vi "User Event LV2 Stop.vi"(0 "Stop":bool=TRUE, 11 "Error In":errorcluster, 13 "Operation":T1) -> (4 "User Event Ref":refnum<user-event>, 15 "Error Out":errorcluster)   [LabVIEW 2023]
doc: "The file is the Functional global to store the user event reference to stop when user clicks panel close."
uses:
  Typedef/User Event Operations.ctl
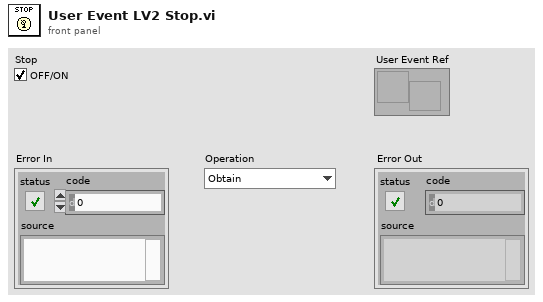
[diagram p1: front panel]
types:
  T1 = typedef "User Event Operations.ctl" = enum16{"Obtain", "Generate", "Release"}
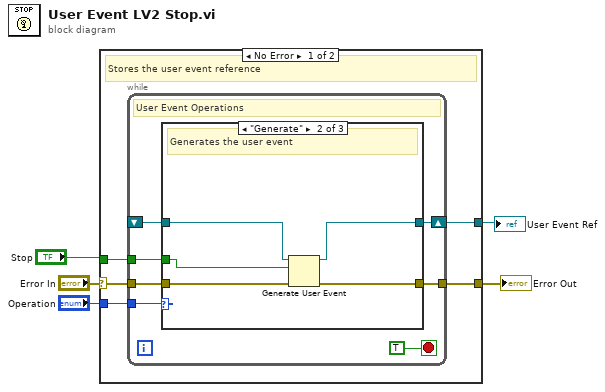
[diagram p0: block diagram]
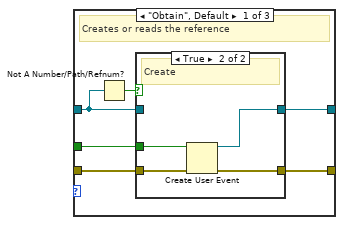
[diagram p2: hidden frame]
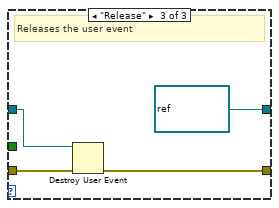
[diagram p4: hidden frame]
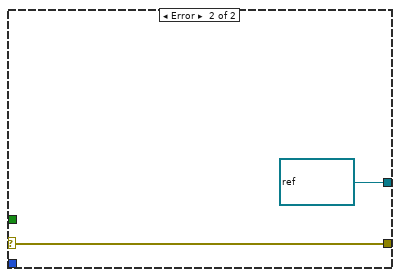
[diagram p5: hidden frame]
diagram:
  n1 = case shown="No Error" "Error In" {
    selector: "Error In" -> [w8 w40]
    tunnel: "Operation" -> [w10 _]
    tunnel: "Stop" -> [w9 _]
    tunnel: [w7 w40] -> w3
    tunnel: [w6 refnum<user-event> refnum ("Data")] -> w1
    frame No Error {
      # "Stores the user event reference"
      n2 = while {
        tunnel: w10 -> [w17]
        tunnel: w9 -> [w16]
        tunnel: w8 -> [w15]
        tunnel: [w14] -> w7
        shift-right: [w13] -> w6
        shift-left: _ -> [w12]
        stop <- TRUE stop-if-true
        # "User Event Operations"
        n3 = case shown="\"Generate\"" w17 {
          tunnel: w16 -> [w21 w34 _]
          tunnel: w15 -> [w22 w33 w37]
          tunnel: [w23 w32 w38] -> w14
          tunnel: [w20 w30 refnum<user-event> refnum ("Data")] -> w13
          tunnel: w12 -> [w19 w31 w36]
          frame "Obtain", Default {
            # "Creates or reads the reference"
            n4 = Not A Number/Path/Refnum?(number/path/refnum=w19) -> (NaN/Path/Refnum?=w18:bool)
            n5 = case shown="True" w18 {
              tunnel: [w24 w29] -> w23
              tunnel: w22 -> [w24 w28]
              tunnel: w21 -> [_ w27]
              tunnel: [w25 w26] -> w20
              tunnel: w19 -> [w25 _]
              frame False {
                # "Use existing"
              }
              frame True {
                # "Create"
                n6 = Create User Event(user event datatype=w27, error in=w28) -> (user event=w26:refnum<user-event>, error out=w29:errorcluster)
              }
            }
          }
          frame "Generate" {
            # "Generates the user event"
            n7 = Generate User Event(user event=w31, event data cluster=w34, error in=w33) -> (user event out=w30:refnum<user-event>, error out=w32:errorcluster)  [unwired: 1 in]
          }
          frame "Release" {
            # "Releases the user event"
            n8 = Destroy User Event(user event=w36, error in=w37) -> (error out=w38:errorcluster)
          }
        }
      }
    }
    frame Error {
    }
  }
  "Error Out" <- w3
  "User Event Ref" <- w1
